vi "FilterDisabledTachometers.vi"(7 "channels enabled":bool[](array[boolean]), 8 "error in (no error)":errorcluster, 10 "Sampling Info":T1={"Number of Channels"=4, "Sampling Rate"=5120.0, "Channels"=[], "Units"=[], "Offsets"=[]}, 11 "Pulse Positions Array in":T2[](array[typedef])) -> (0 "error out":errorcluster, 3 "Pulse Positions Array out":T2[](array[typedef]))   [LabVIEW 2017, in "CmsAcquisition.lvlib"]
uses:
  <vilib>/addons/InsightCM/Devices/Shared/Cms/CmsAcquisition/CmsAcquisition.lvlib
  <vilib>/addons/InsightCM/Utilities/Analysis/Shared/controls/PulsePositions.ctl
  <vilib>/addons/InsightCM/Devices/Shared/Cms/cRIOWfmAcq/subVIs/RIO Wfm Cust Ctrls/rwfm_SamplingInfo.ctl
  <vilib>/addons/InsightCM/Utilities/Analysis/Shared/AnalysisHelper.lvlib
  <vilib>/addons/InsightCM/Devices/Shared/Cms/cRIOWfmAcq/cRIOWfmLib.lvlib
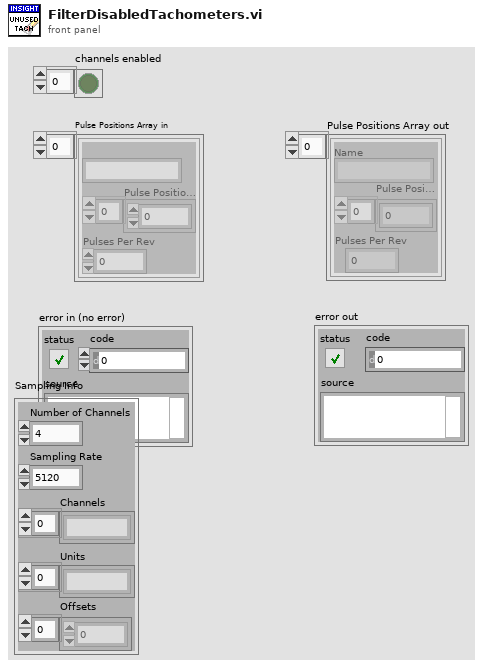
[diagram p1: front panel]
types:
  T1 = typedef "cRIOWfmLib.lvlib/rwfm_SamplingInfo.ctl" = cluster{"Number of Channels":i32, "Sampling Rate":dbl, "Channels":string[], "Units":string[], "Offsets":sgl[]}
  T2 = typedef "AnalysisHelper.lvlib/PulsePositions.ctl" = cluster{"Name":string, "Pulse Position Data":dbl[], "Pulses Per Rev":i32}
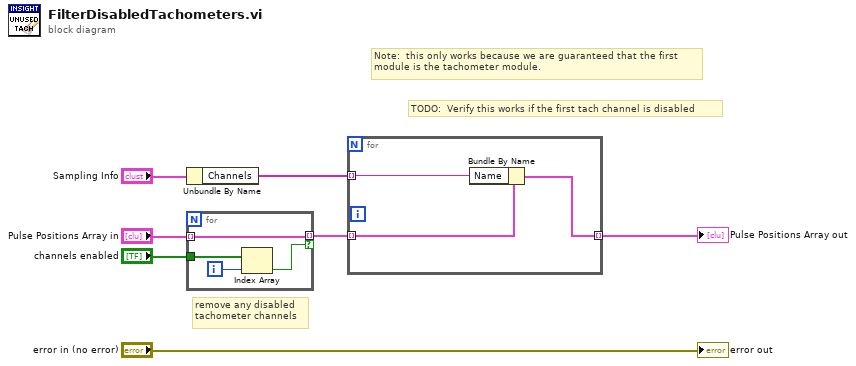
[diagram p0: block diagram]
diagram:
  # "TODO:  Verify this works if the first tach channel is disabled"
  # "Note:  this only works because we are guaranteed that the first\nmodule is the tachometer module."
  # "remove any disabled \ntachometer channels"
  n1 = Unbundle By Name("Sampling Info") -> ("Channels"=w1:string[])
  n2 = for {
    tunnel: "channels enabled" -> [w10]
    tunnel: [w9] -> w3 mode=indexing if=w8
    tunnel: "Pulse Positions Array in" -> [w9] mode=indexing
    i -> [w11]
    n3 = Index Array(array=w10, index=w11) -> (element=w8:bool)
  }
  n4 = for {
    tunnel: [w13] -> w4 mode=indexing
    tunnel: w3 -> [w14] mode=indexing
    tunnel: w1 -> [w12] mode=indexing
    n5 = Bundle By Name(cluster=w14, "Name"=w12) -> (w13:T2)
  }
  "Pulse Positions Array out" <- w4
  "error out" <- "error in (no error)"
